vi "MC5e Calculate Unit.vi"(6 "index":i32, 7 "Mode":T7, 9 "Unit In":T2={"Unit Fatigue Level"=enum."Not Fatigued", "Flying Unit"=FALSE, "Mounted Unit"=FALSE, "Defending from Stronghold"=FALSE, "Difficult Terrain Types"=[0, 1, 3, 6, 7], "Squads in Unit"=[], "Unit Info"={"Unit Name"="", "Unit Commander"="", "Morale Mod"=0, "BR Mod"=0, "Defense Mod"=0, "Speed Mod"=0, "Unit Notes"="", "Attack Mod"=0, "Unit Wins+ Losses-"=0, "Commander Charisma Bonus"=0}, "Range"=0, "BR"=0, "Speed"=0, "Morale"=0, "Current BR"=0, "Location"={"X coordinate"=0.0, "Y coordinate"=0.0}, "Capacity %"=0} {"Squads in Unit"."CR" items=["30", "29", "28", "27", "26", "25", "24", "23", "22", "21", "20", "19", "18", "17", "16", "15", "14", "13", "12", "11", "10", "9", "8", "7", "6", "5", "4", "3", "2", "1", "1/2", "1/4", "1/8"]}, 11 "Unit Info":T1) -> (1 "Unit Out":T2={"Unit Fatigue Level"=enum."Not Fatigued", "Flying Unit"=FALSE, "Mounted Unit"=FALSE, "Defending from Stronghold"=FALSE, "Difficult Terrain Types"=[0, 1, 3, 6, 7], "Squads in Unit"=[], "Unit Info"={"Unit Name"="", "Unit Commander"="", "Morale Mod"=0, "BR Mod"=0, "Defense Mod"=0, "Speed Mod"=0, "Unit Notes"="", "Attack Mod"=0, "Unit Wins+ Losses-"=0, "Commander Charisma Bonus"=0}, "Range"=0, "BR"=0, "Speed"=0, "Morale"=0, "Current BR"=0, "Location"={"X coordinate"=0.0, "Y coordinate"=0.0}, "Capacity %"=0} {"Squads in Unit"."CR" items=["30", "29", "28", "27", "26", "25", "24", "23", "22", "21", "20", "19", "18", "17", "16", "15", "14", "13", "12", "11", "10", "9", "8", "7", "6", "5", "4", "3", "2", "1", "1/2", "1/4", "1/8"]}, 2 "OK Button Disabled?":T8(ring), 3 "Unit Info Out":T1)   [LabVIEW 2020]
uses:
  MC5e Editor modes.ctl
  MC5e Unit Header.ctl
  MC5e Unit.ctl
  MC5e Terrain types.ctl
  MC5e Squad_Info.ctl
  MC5e Size_Categories.ctl
  Location.ctl
  <vilib>/Analysis/baseanly.llb/Mean (DBL).vi
  <vilib>/Analysis/NI_AALBase.lvlib
panel:
  # "Squads are restricted to one type of soldier (i.e  Archers) and all of the same level.\nIf you want mixed CR or mixed types, use multiple squads."
  # "Squads are restricted to one type of soldier (i.e  Archers) and all of the same level.\nIf you want mixed CR or mixed types, use multiple squads."
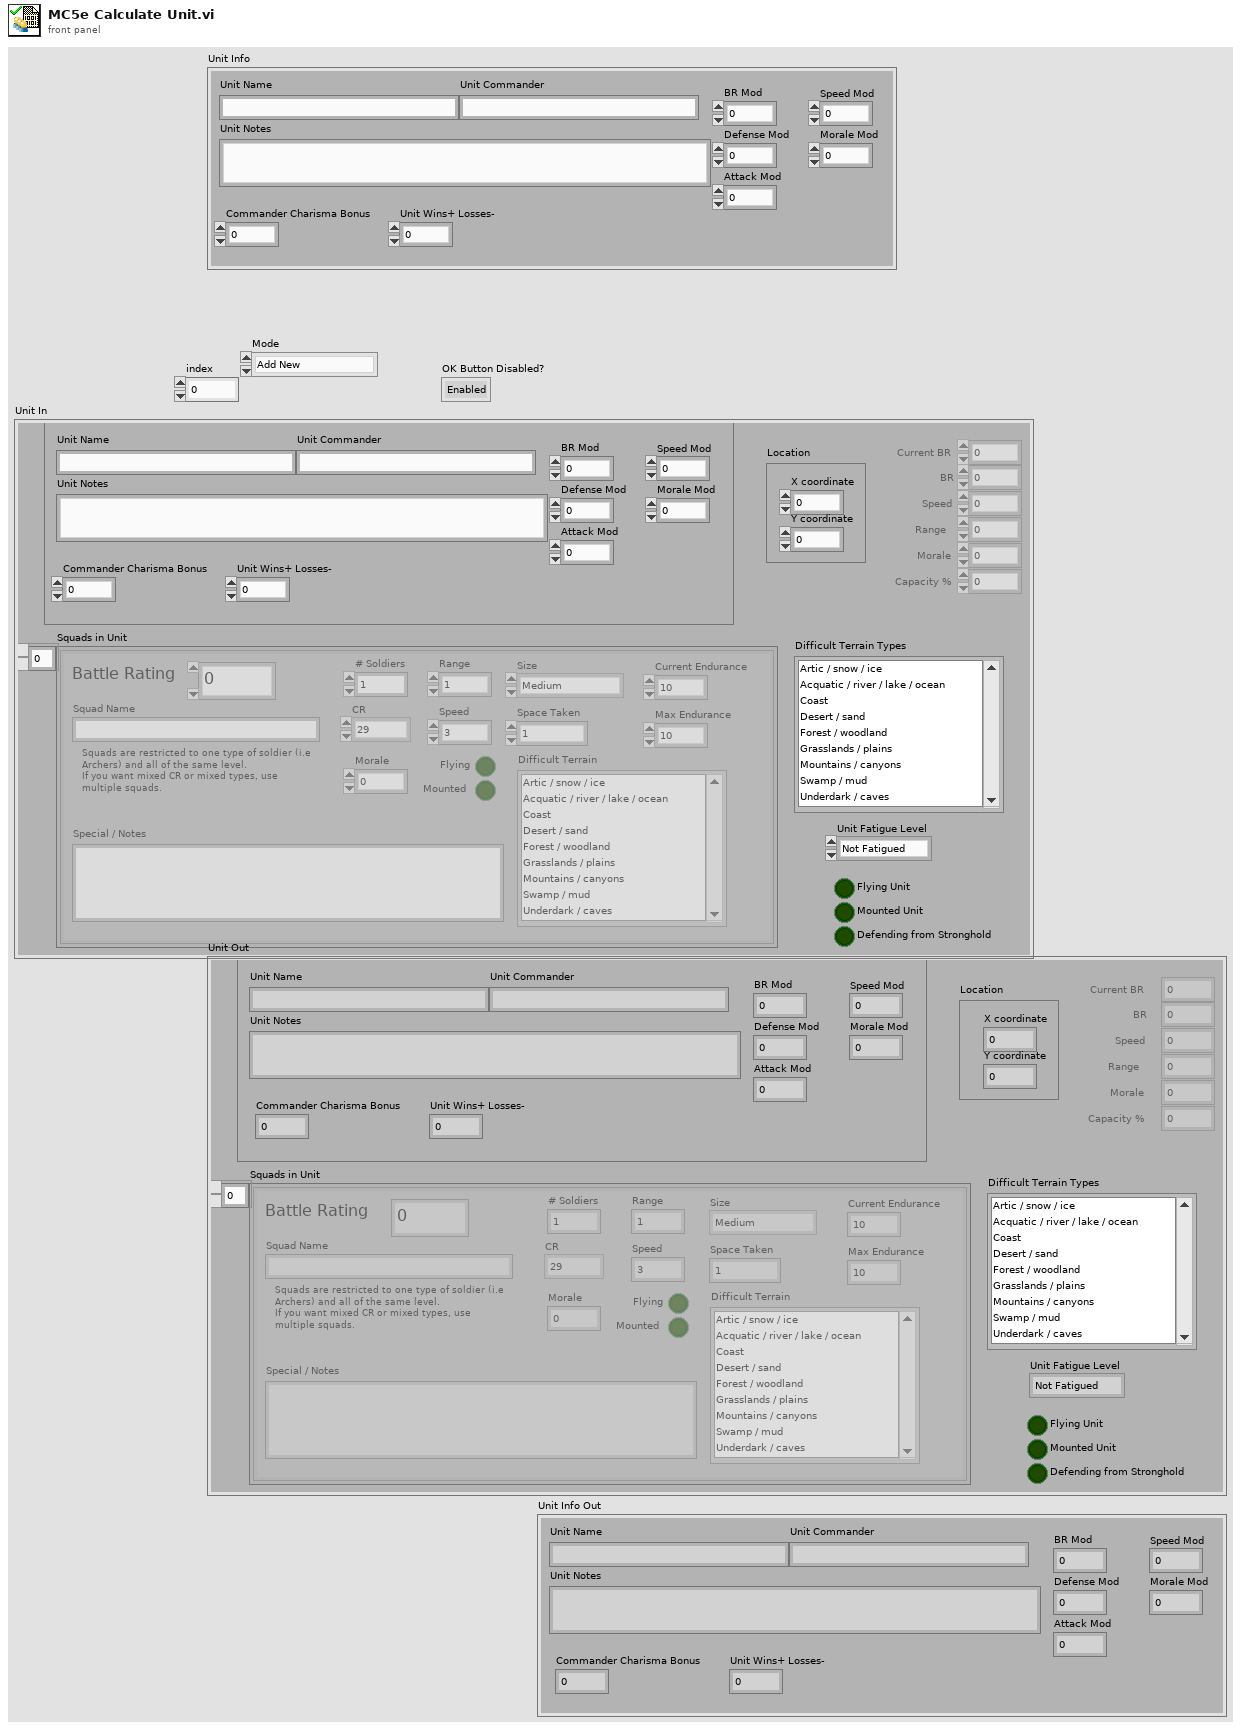
[diagram p1: front panel]
types:
  T1 = typedef "MC5e Unit Header.ctl" = cluster{"Unit Name":string, "Unit Commander":string, "Morale Mod":i32, "BR Mod":i32, "Defense Mod":i32, "Speed Mod":i32, "Unit Notes":string, "Attack Mod":i32, "Unit Wins+ Losses-":i32, "Commander Charisma Bonus":i32}
  T2 = typedef "MC5e Unit.ctl" = cluster{"Unit Fatigue Level":enum16{"Not Fatigued", "Fatigued", "Seriously Fatigued"}, "Flying Unit":bool, "Mounted Unit":bool, "Defending from Stronghold":bool, "Difficult Terrain Types":T3, "Squads in Unit":T4[], "Unit Info":T1, "Range":i32, "BR":i32, "Speed":i32, "Morale":i32, "Current BR":i32, "Location":T6, "Capacity %":i32}
  T3 = typedef "MC5e Terrain types.ctl" = i32[]
  T4 = typedef "MC5e Squad_Info.ctl" = cluster{"Squad Name":string, "# Soldiers":u16, "Battle Rating":u16, "Flying":bool, "Mounted":bool, "Speed":u16, "Range":u16, "Morale":i32, "Max Endurance":u16, "Current Endurance":i32, "Size":T5, "Space Taken":u16, "Difficult Terrain":i32[], "CR":u16, "Special / Notes":string}
  T5 = typedef "MC5e Size_Categories.ctl" = enum16{"Tiny", "Small", "Medium", "Large", "Huge", "Gargantuan"}
  T6 = typedef "Location.ctl" = cluster{"X coordinate":dbl, "Y coordinate":dbl}
  T7 = typedef "MC5e Editor modes.ctl" = enum16{"Add New", "Copy Selected", "Delete Selected", "Edit Selected"}
  T8 = enum8{"Enabled", "Disabled", "Disabled and Grayed Out"}
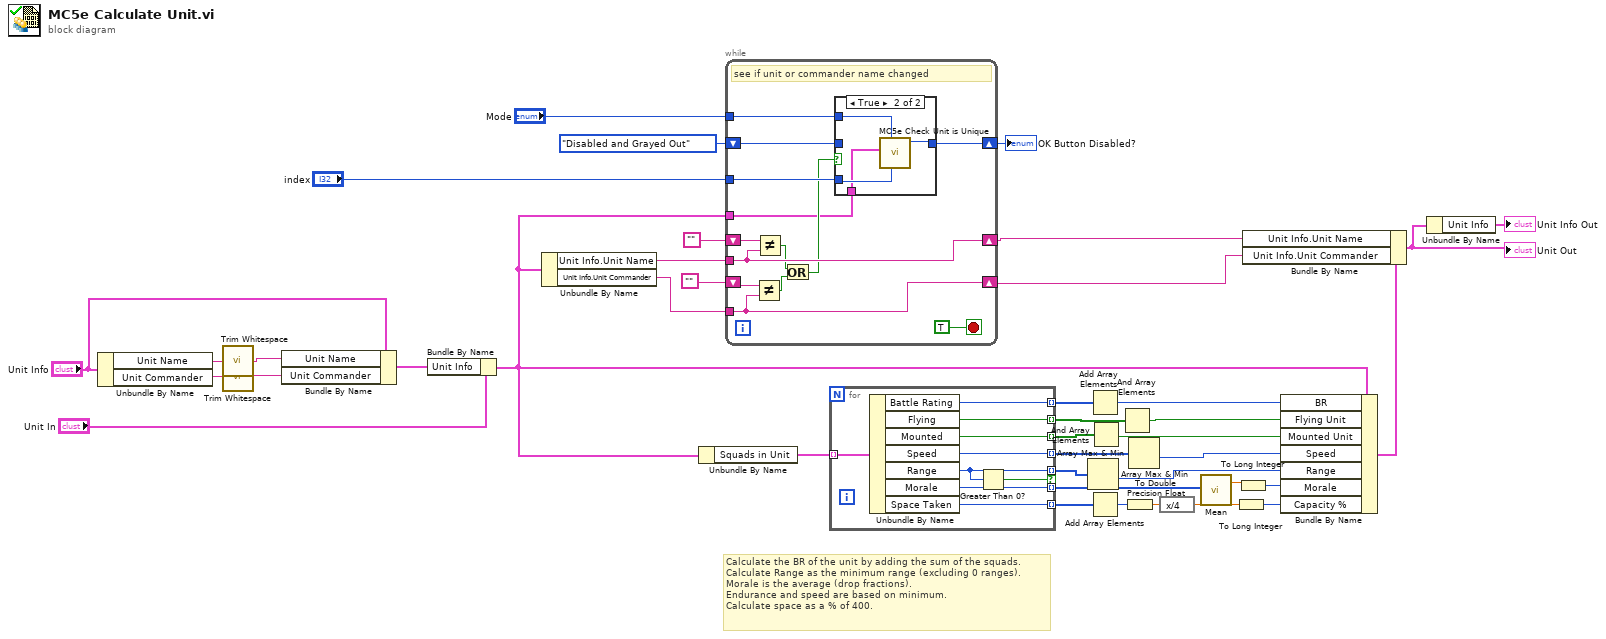
[diagram p0: block diagram]
diagram:
  # "Calculate the BR of the unit by adding the sum of the squads.\nCalculate Range as the minimum range (excluding 0 ranges).\nMorale is the average (drop fractions).\nEndurance and speed are based on minimum.\nCalculate space as a % of 400."
  n1 = Unbundle By Name("Unit Info") -> ("Unit Name"=w30:string, "Unit Commander"=w29:string)
  n2 = call <vilib>:"Trim Whitespace.vi"("string"=w30) -> ("trimmed string"=w4:string)  [unwired: 1 in]
  n3 = call <vilib>:"Trim Whitespace.vi"("string"=w29) -> ("trimmed string"=w6:string)  [unwired: 1 in]
  n4 = Bundle By Name(cluster="Unit Info", "Unit Name"=w4, "Unit Commander"=w6) -> (w5:T1)
  n5 = Bundle By Name(cluster="Unit In", "Unit Info"=w5) -> (w3:T2)
  n6 = Unbundle By Name(w3) -> ("Unit Info.Unit Name"=w2:string, "Unit Info.Unit Commander"=w1:string)
  n7 = Unbundle By Name(w3) -> ("Squads in Unit"=w27:T4[])
  n8 = while {
    shift-right: [w51] -> w34
    shift-left: "" -> [w52]
    tunnel: w2 -> [w51]
    shift-right: [w50] -> w39
    shift-left: T8."Disabled and Grayed Out" ("OK Button Disabled?") -> [w49]
    tunnel: "index" -> [w48]
    tunnel: "Mode" -> [w47]
    shift-right: [w45] -> w33
    shift-left: "" -> [w46]
    tunnel: w1 -> [w45]
    tunnel: w3 -> [w41]
    stop <- TRUE stop-if-true
    # "see if unit or commander name changed"
    n9 = Not Equal?(x=w46, y=w45) -> (x != y?=w44:bool)
    n10 = Not Equal?(x=w52, y=w51) -> (x != y?=w43:bool)
    n11 = Or(x=w43, y=w44) -> (x .or. y?=w42:bool)
    n12 = case shown="True" w42 {
      tunnel: [w54 w58] -> w50
      tunnel: w49 -> [w54 _]
      tunnel: w48 -> [_ w57]
      tunnel: w47 -> [_ w56]
      tunnel: w41 -> [_ w55]
      frame False {
      }
      frame True {
        n13 = call "MC5e Check Unit is Unique.vi"("index"=w57, "Mode"=w56, "Unit"=w55) -> ("OK Button Disabled?"=w58:T8)  [unwired: 6 in, 2 out]
      }
    }
  }
  "OK Button Disabled?" <- w39
  n14 = for {
    tunnel: w27 -> [w67] mode=indexing
    tunnel: [w66] -> w26 mode=indexing
    tunnel: [w65] -> w24 mode=indexing
    tunnel: [w64] -> w22 mode=indexing
    tunnel: [w63] -> w19 mode=indexing
    tunnel: [w62] -> w17 mode=indexing if=w61
    tunnel: [w60] -> w15 mode=indexing
    tunnel: [w59] -> w12 mode=indexing
    n15 = Unbundle By Name(w67) -> ("Battle Rating"=w66:u16, "Flying"=w65:bool, "Mounted"=w64:bool, "Speed"=w63:u16, "Range"=w62:u16, "Morale"=w60:i32, "Space Taken"=w59:u16)
    n16 = Greater Than 0?(x=w62) -> (x > 0?=w61:bool)
  }
  n17 = Array Max & Min(array=w17) -> (min value=w16:u16)  [unwired: 3 out]
  n18 = Add Array Elements(numeric array=w26) -> (sum=w25:u16)
  n19 = Add Array Elements(numeric array=w12) -> (sum=w11:u16)
  n20 = And Array Elements(Boolean array=w22) -> (logical AND=w21:bool)
  n21 = And Array Elements(Boolean array=w24) -> (logical AND=w23:bool)
  n22 = To Double Precision Float(number=w11) -> (double precision float=w9:dbl)
  n23 = Array Max & Min(array=w19) -> (min value=w18:u16)  [unwired: 3 out]
  n24 = expression code="x/4"(w9) -> (w10:dbl)
  n25 = call-poly <vilib>:"Mean.vi"("X"=w15) -> ("mean"=w14:dbl)  [unwired: 1 out]
  n26 = To Long Integer(number=w10) -> (32bit integer=w8:i32)
  n27 = To Long Integer(number=w14) -> (32bit integer=w13:i32)
  n28 = Bundle By Name(cluster=w3, "BR"=w25, "Flying Unit"=w23, "Mounted Unit"=w21, "Speed"=w18, "Range"=w16, "Morale"=w13, "Capacity %"=w8) -> (w20:T2)
  n29 = Bundle By Name(cluster=w20, "Unit Info.Unit Name"=w34, "Unit Info.Unit Commander"=w33) -> (w32:T2)
  "Unit Out" <- w32
  n30 = Unbundle By Name(w32) -> ("Unit Info"=→"Unit Info Out":T1)
